vi "Close P1 P2 Factor DVRs.vi"(10 "P2 Factors DVR":refnum<data-value>, 11 "P1 Factors DVR":refnum<data-value>) -> (0 "error out":errorcluster)   [LabVIEW 2013]
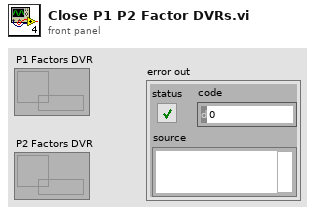
[diagram p1: front panel]
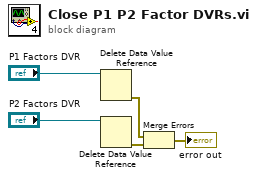
[diagram p0: block diagram]
diagram:
  n1 = Delete Data Value Reference(data value reference="P1 Factors DVR") -> (error out=w2:errorcluster)  [unwired: 1 in, 1 out]
  n2 = Delete Data Value Reference(data value reference="P2 Factors DVR") -> (error out=w3:errorcluster)  [unwired: 1 in, 1 out]
  n3 = Merge Errors(w2, w3) -> (→"error out":errorcluster)
